vi "Roller Speed Control.vi"(9 "From shift":dbl format="%#_13g", 10 "Off?":bool, 11 "Roller speed(raw)":dbl) -> (2 "To shift":dbl format="%#_13g", 3 "Motor Output":dbl)   [LabVIEW 2013]
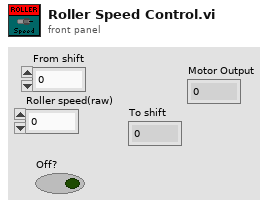
[diagram p1: front panel]
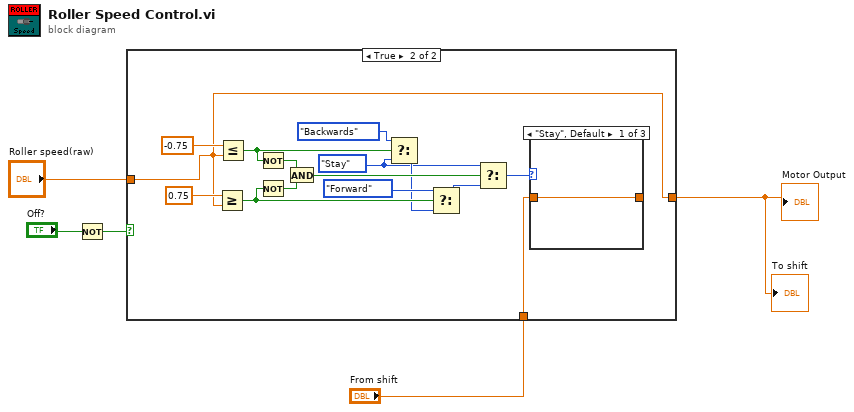
[diagram p0: block diagram]
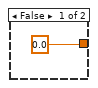
[diagram p2: hidden frame]
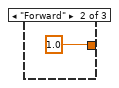
[diagram p3: hidden frame]
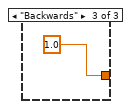
[diagram p4: hidden frame]
diagram:
  n1 = Not(x="Off?") -> (.not. x?=w2:bool)
  n2 = case shown="True" w2 {
    tunnel: "Roller speed(raw)" -> [_ w7]
    tunnel: "From shift" -> [_ w8]
    tunnel: [0.0 w7] -> w3
    frame False {
    }
    frame True {
      w10 = enum16{"Stay", "Forward", "Backwards"}."Stay"
      n3 = Greater Or Equal?(x=0.75, y=w7) -> (x >= y?=w14:bool)
      n4 = Less Or Equal?(x=-0.75, y=w7) -> (x <= y?=w11:bool)
      n5 = Not(x=w11) -> (.not. x?=w19:bool)
      n6 = Not(x=w14) -> (.not. x?=w18:bool)
      n7 = And(x=w19, y=w18) -> (x .and. y?=w17:bool)
      n8 = Select(t=enum16{"Stay", "Forward", "Backwards"}."Backwards", s=w11, f=w10) -> (s? t:f=w12:enum16{"Stay", "Forward", "Backwards"})
      n9 = Select(t=enum16{"Stay", "Forward", "Backwards"}."Forward", s=w14, f=w12) -> (s? t:f=w15:enum16{"Stay", "Forward", "Backwards"})
      n10 = Select(t=w10, s=w17, f=w15) -> (s? t:f=w16:enum16{"Stay", "Forward", "Backwards"})
      n11 = case shown="\"Stay\", Default" w16 {
        tunnel: [w22 1.0 1.0] -> _
        tunnel: w8 -> [w22 _ _]
        frame "Stay", Default {
        }
        frame "Forward" {
        }
        frame "Backwards" {
        }
      }
    }
  }
  "To shift" <- w3
  "Motor Output" <- w3
